vi "Set Ext Trigger Mode.vi"(7 "Ref Trigger Mode":refnum<vi>, 8 "error in":errorcluster, 10 "Pulsar Handle":i16, 11 "OphirFastX (in)":refnum<k7>) -> (0 "error out":errorcluster, 3 "OphirFastX (out)":refnum<k7>)   [LabVIEW 2009]
panel:
  # "Guillaume Plateau - yguig2@yahoo.fr"
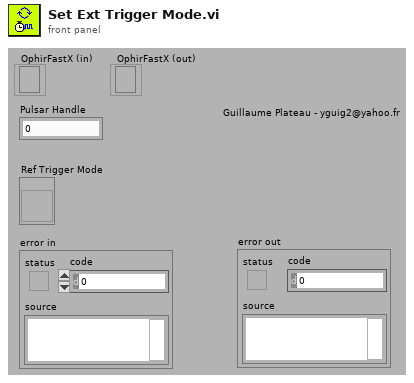
[diagram p1: front panel]
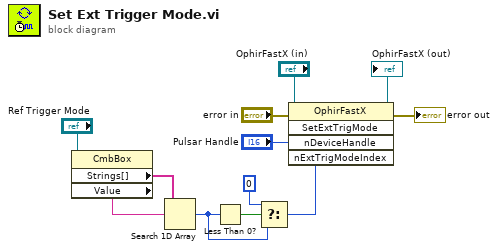
[diagram p0: block diagram]
diagram:
  n1 = property class="CmbBox"(reference="Ref Trigger Mode") -> ("Strings[]"=w9:string[], "Value"=w3:string)  [unwired: 1 in, 2 out]
  n2 = Search 1D Array(1D array=w9, element=w3) -> (index of element=w6:i32)  [unwired: 1 in]
  n3 = Less Than 0?(x=w6) -> (x < 0?=w8:bool)
  n4 = Select(t=i16 0 ("nRangeIndex"), s=w8, f=w6) -> (s? t:f=w4:i32)
  n5 = invoke class="OphirFastX" method="SetExtTrigMode"(reference="OphirFastX (in)", error in="error in", "nDeviceHandle"="Pulsar Handle", "nExtTrigModeIndex"=w4) -> (reference out=→"OphirFastX (out)":refnum<k7>, error out=→"error out":errorcluster)  [unwired: 1 in, 3 out]
